vi "Calibrate.vi"() -> ()   [LabVIEW 2020]
uses:
  Classes/Controller/Controller.lvclass
  Classes/Assembly/Calibrate/Calibrate.lvclass
  Classes/Module/Module.lvclass
panel:
  in  "Component Tray Number":i32
  in  "Stage":i32(listbox)
  in  "Go":bool
  in  "Position Number":i32
  in  "Assembly Tray Number":i32
  in  "Assembly Tray Region":i32
  in  "Stop":bool
  in  "Build":bool
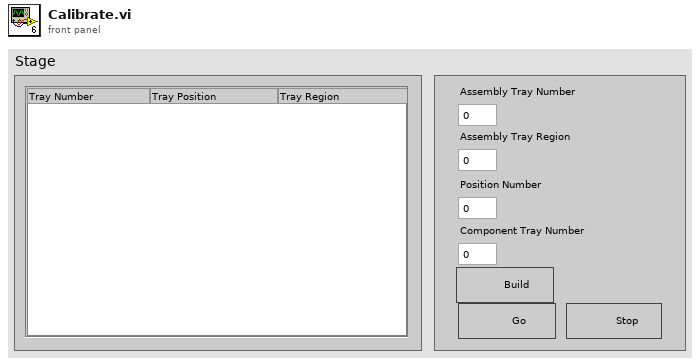
[diagram p1: front panel]
types:
  T1 = typedef "Controller.lvclass/Controllers.ctl" = cluster{"I-O.lvclass":refnum<class "I-O.lvclass">, "Gantry":refnum<k24>, "Dispenser":refnum<visa-resource-name>}
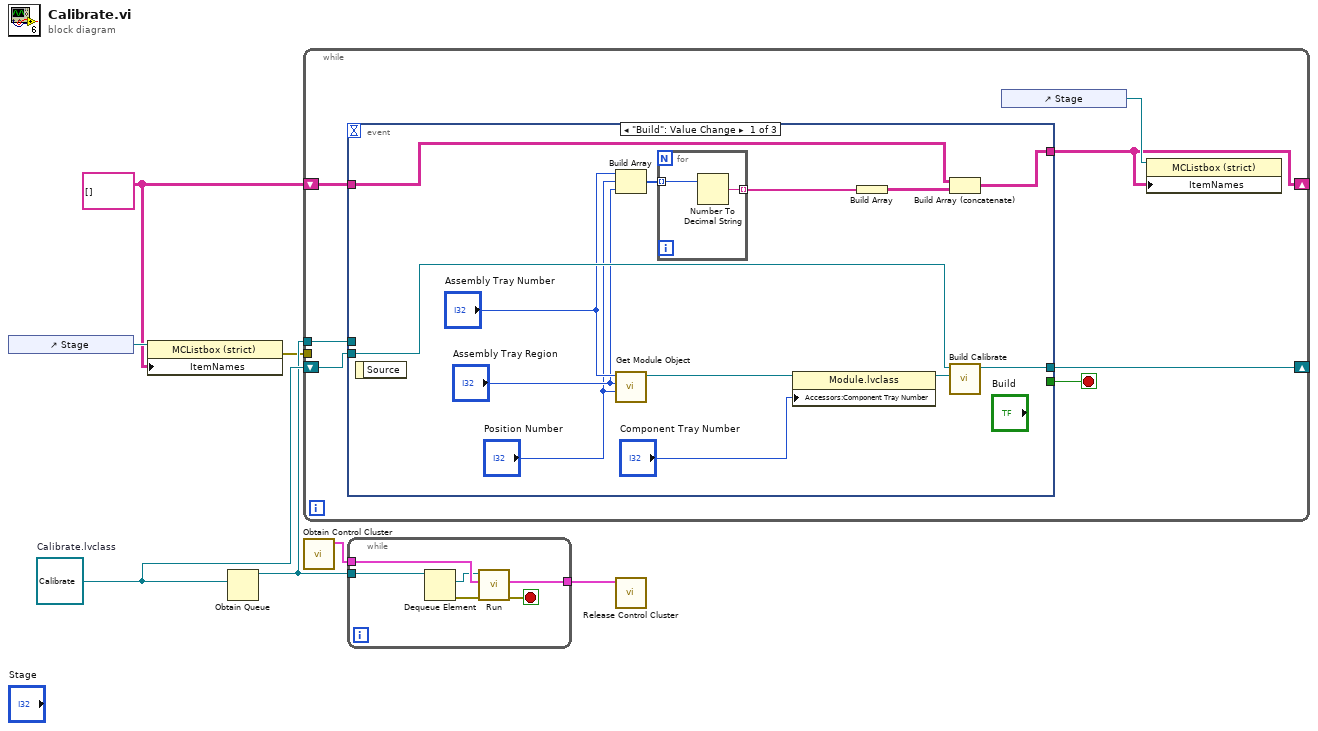
[diagram p0: block diagram]
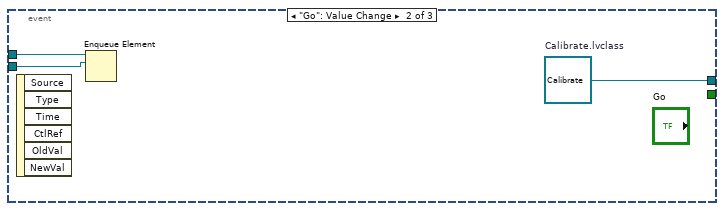
[diagram p2: hidden frame]
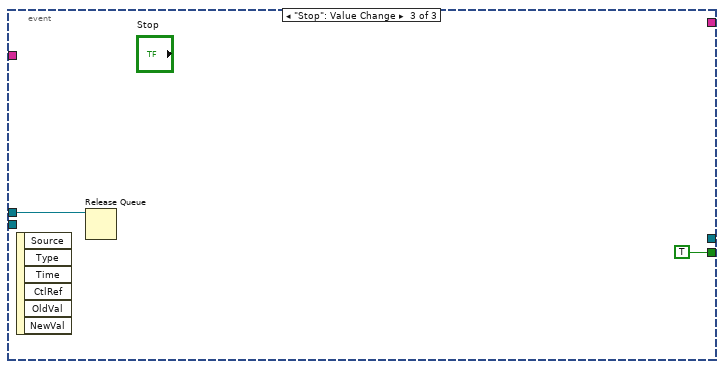
[diagram p3: hidden frame]
diagram:
  w2 = string[][] [] ("element")
  w5 = refnum<class "Calibrate.lvclass"> refnum  # Calibrate.lvclass
  n1 = control-ref of="Stage"() -> (w3:refnum<vi>)
  n2 = property class="MCListbox (strict)"(reference=w3, "ItemNames"=w2) -> (error out=w1:errorcluster)  [unwired: 1 in, 1 out]
  n3 = Obtain Queue(element data type=w5) -> (queue out=w4:refnum<queue>)  [unwired: 4 in, 2 out]
  n4 = while {
    tunnel: w4 -> [w13]
    shift-right: [w11] -> _
    shift-left: w5 -> [w14]
    shift-right: [w8] -> _
    shift-left: w2 -> [w9]
    tunnel: w1 -> [_]
    stop <- w12 stop-if-true
    n5 = event shown="[0] \"Build\": Value Change" {
      selector: _ -> [_ _ _]
      dyn-events: _ -> [_ _ _]
      timeout: _ -> [_ _ _]
      tunnel: w14 -> [w27 w31 _]
      tunnel: w13 -> [_ w32 w33]
      tunnel: [_ _ TRUE] -> w12
      tunnel: [w26 w30 _] -> w11
      tunnel: [w18 _ _] -> w8
      tunnel: w9 -> [w19 _ _]
      event "Build": Value Change {
        n6 = event-data() -> ()  [unwired: 1 in, 1 out]
        n7 = Build Array("Assembly Tray Number", "Position Number", "Assembly Tray Region") -> (w24:i32[])
        n8 = call "Get Module Object.vi"("Assembly Tray Position"="Position Number", "Assembly Tray Region"="Assembly Tray Region", "Assembly Tray Number"="Assembly Tray Number") -> ("Module.lvclass"=w17:refnum<class "Module.lvclass">)  [unwired: 7 in, 1 out]
        n9 = for {
          tunnel: w24 -> [w29] mode=indexing
          tunnel: [w28] -> w23 mode=indexing
          n10 = Number To Decimal String(number=w29) -> (decimal integer string=w28:string)  [unwired: 1 in]
        }
        n11 = property class="Module.lvclass"(reference=w17, "Accessors:Component Tray Number"="Component Tray Number") -> (reference out=w15:refnum<class "Module.lvclass">)  [unwired: 1 in, 1 out]
        n12 = Build Array(w23) -> (w20:string[][])
        n13 = Build Array (concatenate)(w19, w20) -> (w18:string[][])
        n14 = call "Build Calibrate.vi"("Module.lvclass"=w15, "Calibrate in"=w27) -> ("Calibrate out"=w26:refnum<class "Calibrate.lvclass">)  [unwired: 8 in, 1 out]
      }
      event "Go": Value Change {
        w30 = refnum<class "Calibrate.lvclass"> refnum  # Calibrate.lvclass
        n15 = event-data() -> ()  [unwired: 1 in, 6 out]
        n16 = Enqueue Element(queue=w32, element=w31) -> ()  [unwired: 2 in, 3 out]
      }
      event "Stop": Value Change {
        n17 = event-data() -> ()  [unwired: 1 in, 6 out]
        n18 = Release Queue(queue=w33) -> ()  [unwired: 2 in, 3 out]
      }
    }
    n19 = control-ref of="Stage"() -> (w10:refnum<vi>)
    n20 = property class="MCListbox (strict)"(reference=w10, "ItemNames"=w8) -> ()  [unwired: 1 in, 2 out]
  }
  n21 = call "Obtain Control Cluster.vi"() -> ("Control Out"=w6:T1)  [unwired: 11 in]
  n22 = while {
    tunnel: [w40] -> w7
    tunnel: w6 -> [w39]
    tunnel: w4 -> [w38]
    stop <- w35 stop-if-true
    n23 = Dequeue Element(queue=w38) -> (element=w37:refnum<class "Calibrate.lvclass">, error out=w36:errorcluster)  [unwired: 2 in, 2 out]
    n24 = call-dynamic "Run.vi"("error in (no error)"=w36, "Control In"=w39, "Assembly In"=w37) -> ("error out"=w35:errorcluster, "Control Out"=w40:T1)  [unwired: 6 in, 1 out]
  }
  n25 = call "Release Control Cluster.vi"("output cluster"=w7) -> ()  [unwired: 11 in]
